vi "Handle Missing Sections.vi"(6 "any found?":bool, 7 "Section Formatted Cluster In":variant, 8 "error in (no error)":errorcluster, 9 "all found?":bool, 10 "Section Formatted Cluster in":variant, 11 "Refnum in":T1) -> (0 "error out":errorcluster, 2 "Section Formatted Cluster out":variant, 3 "Refnum out":T1)   [LabVIEW 2019, in "Configuration.lvclass"]
uses:
  Configuration.lvclass
  <vilib>/Utility/config.llb/Config Data RefNum.ctl
  <vilib>/Utility/config.llb/NI_LVConfig.lvlib
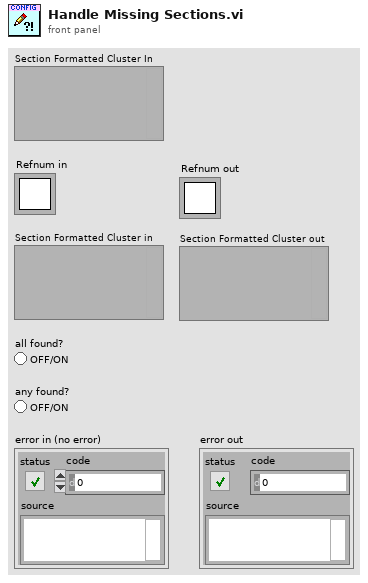
[diagram p1: front panel]
types:
  T1 = typedef "NI_LVConfig.lvlib/Config Data RefNum.ctl" = refnum<k1>
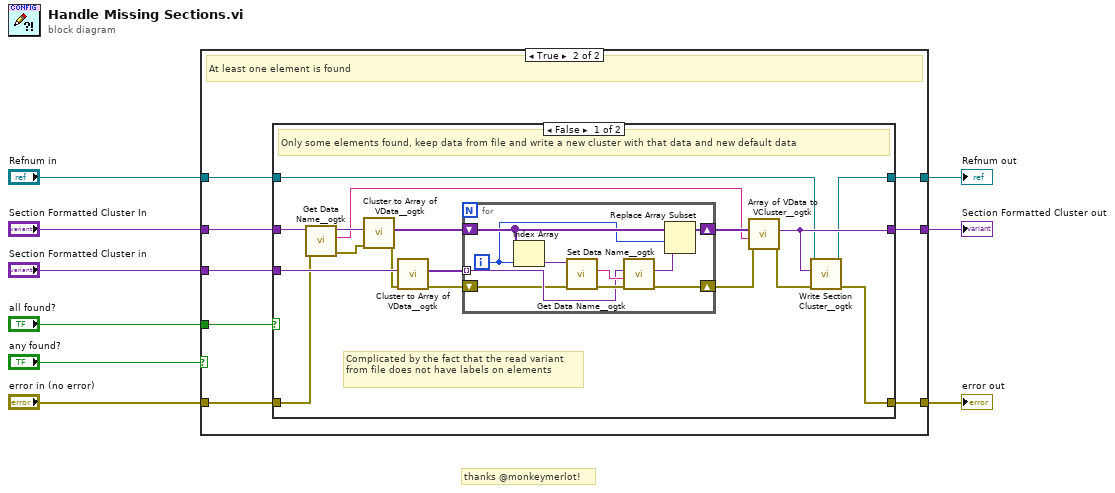
[diagram p0: block diagram]
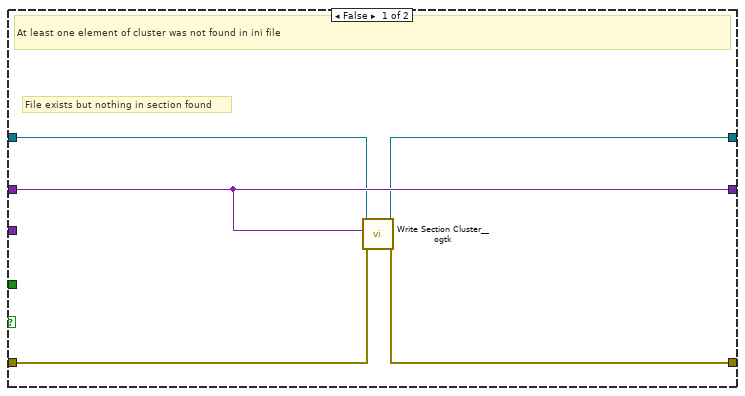
[diagram p2: hidden frame]
diagram:
  # "thanks @monkeymerlot!"
  n1 = case shown="True" "any found?" {
    tunnel: "Section Formatted Cluster In" -> [w14 w15]
    tunnel: "Section Formatted Cluster in" -> [_ w20]
    tunnel: "Refnum in" -> [w10 w19]
    tunnel: [w11 w16] -> w5
    tunnel: [w14 w18] -> w6
    tunnel: "error in (no error)" -> [w13 w21]
    tunnel: [w12 w17] -> w8
    tunnel: "all found?" -> [_ w22]
    frame False {
      # "File exists but nothing in section found"
      # "At least one element of cluster was not found in ini file"
      n2 = call <userlib>:"Write Section Cluster__ogtk.vi"("error in (no error)"=w13, "Section Formatted Cluster"=w14, "refnum"=w10) -> ("error out"=w12:errorcluster, "dup refnum"=w11:T1)  [unwired: 7 in]
    }
    frame True {
      # "At least one element is found"
      n3 = case shown="False" w22 {
        tunnel: w21 -> [w28 w51]
        tunnel: w20 -> [w38 w52]
        tunnel: w19 -> [w24 w50]
        tunnel: [w33 w52] -> w18
        tunnel: [w39 w51] -> w17
        tunnel: [w23 w50] -> w16
        tunnel: w15 -> [w31 _]
        frame False {
          # "Complicated by the fact that the read variant from file does not have labels on elements"
          # "Only some elements found, keep data from file and write a new cluster with that data and new default data"
          n4 = call <userlib>:"Get Data Name__ogtk.vi"("error in (no error)"=w28, "Data"=w31) -> ("error out"=w29:errorcluster, "Data Name"=w30:string, "Data dup"=w32:variant)  [unwired: 7 in]
          n5 = call <userlib>:"Cluster to Array of VData__ogtk.vi"("error in (no error)"=w29, "Cluster"=w32) -> ("error out"=w37:errorcluster, "Array of VData"=w36:variant[])  [unwired: 8 in]
          n6 = call <userlib>:"Cluster to Array of VData__ogtk.vi"("error in (no error)"=w37, "Cluster"=w38) -> ("error out"=w27:errorcluster, "Array of VData"=w35:variant[])  [unwired: 8 in]
          n7 = for {
            tunnel: w35 -> [w42] mode=indexing
            shift-right: [w49] -> w34
            shift-left: w36 -> [w48]
            shift-right: [w40] -> w26
            shift-left: w27 -> [w41]
            i -> [w47]
            n8 = Index Array(array=w48, index=w47) -> (element=w46:variant)
            n9 = call <userlib>:"Get Data Name__ogtk.vi"("error in (no error)"=w41, "Data"=w46) -> ("error out"=w43:errorcluster, "Data Name"=w44:string)  [unwired: 7 in, 1 out]
            n10 = call <userlib>:"Set Data Name__ogtk.vi"("error in (no error)"=w43, "Data Name"=w44, "Data"=w42) -> ("error out"=w40:errorcluster, "Renamed Data"=w45:variant)  [unwired: 7 in]
            n11 = Replace Array Subset(array=w48, new element=w45, index=w47) -> (w49:variant[])
          }
          n12 = call <userlib>:"Array of VData to VCluster__ogtk.vi"("error in (no error)"=w26, "Cluster Name"=w30, "Array"=w34) -> ("error out"=w25:errorcluster, "VCluster"=w33:variant)  [unwired: 7 in]
          n13 = call <userlib>:"Write Section Cluster__ogtk.vi"("error in (no error)"=w25, "Section Formatted Cluster"=w33, "refnum"=w24) -> ("error out"=w39:errorcluster, "dup refnum"=w23:T1)  [unwired: 7 in]
        }
        frame True {
          # "All elements found, use read data"
        }
      }
    }
  }
  "error out" <- w8
  "Section Formatted Cluster out" <- w6
  "Refnum out" <- w5
